vi "GUI.vi"() -> ()   [LabVIEW 2021]
panel:
  in  "Connection Type":u16(ring) items=["USB", "Ethernet"]
  in  "U6 Address":string="192.168.1.199"
  out "POWER\nDISCONNECTED":bool
  in  "?":bool
  in  "SV6":bool
  in  "SV5":bool
  in  "SV4":bool
  in  "START/STOP DATA LOGGING":bool
  in  "SHUTOFF POWER":bool
  in  "SHUTDOWN\nAPPROVE":bool
  in  "SV3":bool
  in  "SV2":bool
  in  "SV1":bool
  in  "SV0":bool
  out "ABORT\nACTIVATED":bool
  out "OVER TEMPERATURE":bool
  out "OVER\nPRESSURE":bool
  in  "GUITabs":T1(tab) caption="Tab Control"
  out "N2O Runtank [g/s]":i16(slide) scale=0.0..100.0
  out "Ethanol Runtank [g/s]":i16(slide) scale=0.0..100.0
  out "?":bool
  out "?":bool
  out "?":bool
  out "LabJack Supply Voltage":dbl(slide) scale=0.0..5.0
  out "Solenoid Supply Voltage":dbl(slide) scale=0.0..14.0
  out "Relay Supply Voltage":dbl(slide) scale=0.0..5.0
  out "PT3: Chamber Pressure [psig]":u16(knob) scale=0.0..500.0
  in  "Arm Button":bool
  in  "Fire Button":bool
  out "DEADMAN\nSWITCH":bool
  out "TC1: N2O Temp [°C]":i16(slide) scale=-270.0..370.0
  out "TC2: Chamber Temp [°C]":i16(slide) scale=-270.0..1260.0
  out "PT1: N2O Pressure [psig]":u16(knob) scale=0.0..1000.0
  out "PT2: Ethenol Pressure [psig]":u16(knob) scale=0.0..1000.0
  out "?":bool
  out "?":bool
  out "Thrust Reading [N]":dbl(slide) scale=0.0..200.0
  in  "Dry Test Run":bool
  in  "Valve\nDiagnostic":bool
  in  "Device\nDiagnostic":bool
  out "?":bool
  out "?":bool
  out "?":bool
  out "?":bool
  out "?":bool
  out "?":bool
  out "?":bool
  out "?":bool
  out "?":bool
  out "?":bool
  out "?":bool
  out "?":bool
  out "?":bool
  in  "S: NC/NO 7":bool
  in  "SV0 Pin":u16(ring)=8 items=["FIO0", "FIO1", "FIO2", "FIO3", "FIO4", "FIO5", "FIO6", "FIO7", "EIO0", "EIO1", "EIO2", "EIO3", "EIO4", "EIO5", "EIO6", "EIO7", "CIO0", "CIO1", "CIO2", "CIO3", "MIO0", "MIO1", "MIO2"]
  in  "SV1":u16(ring)=9 items=["FIO0", "FIO1", "FIO2", "FIO3", "FIO4", "FIO5", "FIO6", "FIO7", "EIO0", "EIO1", "EIO2", "EIO3", "EIO4", "EIO5", "EIO6", "EIO7", "CIO0", "CIO1", "CIO2", "CIO3", "MIO0", "MIO1", "MIO2"]
  in  "SV3 Pin":u16(ring)=11 items=["FIO0", "FIO1", "FIO2", "FIO3", "FIO4", "FIO5", "FIO6", "FIO7", "EIO0", "EIO1", "EIO2", "EIO3", "EIO4", "EIO5", "EIO6", "EIO7", "CIO0", "CIO1", "CIO2", "CIO3", "MIO0", "MIO1", "MIO2"]
  in  "SV2 Pin":u16(ring)=10 items=["FIO0", "FIO1", "FIO2", "FIO3", "FIO4", "FIO5", "FIO6", "FIO7", "EIO0", "EIO1", "EIO2", "EIO3", "EIO4", "EIO5", "EIO6", "EIO7", "CIO0", "CIO1", "CIO2", "CIO3", "MIO0", "MIO1", "MIO2"]
  in  "SV6 Pin":u16(ring)=14 items=["FIO0", "FIO1", "FIO2", "FIO3", "FIO4", "FIO5", "FIO6", "FIO7", "EIO0", "EIO1", "EIO2", "EIO3", "EIO4", "EIO5", "EIO6", "EIO7", "CIO0", "CIO1", "CIO2", "CIO3", "MIO0", "MIO1", "MIO2"]
  in  "SV5 Pin":u16(ring)=13 items=["FIO0", "FIO1", "FIO2", "FIO3", "FIO4", "FIO5", "FIO6", "FIO7", "EIO0", "EIO1", "EIO2", "EIO3", "EIO4", "EIO5", "EIO6", "EIO7", "CIO0", "CIO1", "CIO2", "CIO3", "MIO0", "MIO1", "MIO2"]
  in  "SV4 Pin":u16(ring)=12 items=["FIO0", "FIO1", "FIO2", "FIO3", "FIO4", "FIO5", "FIO6", "FIO7", "EIO0", "EIO1", "EIO2", "EIO3", "EIO4", "EIO5", "EIO6", "EIO7", "CIO0", "CIO1", "CIO2", "CIO3", "MIO0", "MIO1", "MIO2"]
  in  "S: NC/NO 6":bool
  in  "S: NC/NO 5":bool
  in  "S: NC/NO 4":bool
  in  "S: NC/NO 3":bool
  in  "S: NC/NO 2":bool=TRUE
  in  "S: NC/NO":bool=TRUE
  in  "R: NC/NO 7":bool=TRUE
  in  "R: NC/NO 6":bool=TRUE
  in  "R: NC/NO 5":bool=TRUE
  in  "R: NC/NO 4":bool=TRUE
  in  "R: NC/NO 3":bool=TRUE
  in  "R: NC/NO 2":bool=TRUE
  in  "R: NC/NO":bool=TRUE
  in  "?":bool
  in  "TC1 Type":u16(ring)=7 items=["B", "E", "J", "K", "N", "R", "S", "T"]
  in  "TC2 Type":u16(ring)=3 items=["B", "E", "J", "K", "N", "R", "S", "T"]
  in  "TC1 +Channel":u16
  in  "TC2 -Channel":u16=3
  in  "TC2 +Channel":u16=2
  in  "TC1 -Channel":u16=1
  in  "PT2 Pin":u16=6
  in  "PT1 Pin":u16=8
  in  "PT3 Pin":u16=4
  in  "LP1 Pin":u16=10
  in  "k":dbl=2000.0
  # "ABORT STATUS"
  # "MANUAL DATA CONTROL"
  # "OVERRIDE SYSTEM POWER"
  # "LABJACK CONNECTION"
  # "LINE & CHAMBER STATUS"
  # "HIL TEST PARAMETERS"
  # "SYSTEM FIRE OPERATION"
  # "SYSTEM TEST SEQUENCE"
  # "THRUST STATUS"
  # "RUNTANK STATUS"
  # "SYSTEM ERROR CALLSTACK"
  # "DATA LOGGING"
  # "PRESSURE TRANSMITTER SETTINGS"
  # "THERMOCOUPLE SETTINGS"
  # "SOLENOID VALVE & RELAY SETTINGS"
  # "CALIBRATION SETTINGS"
  # "LINEAR POTENTIOMETER SETTINGS"
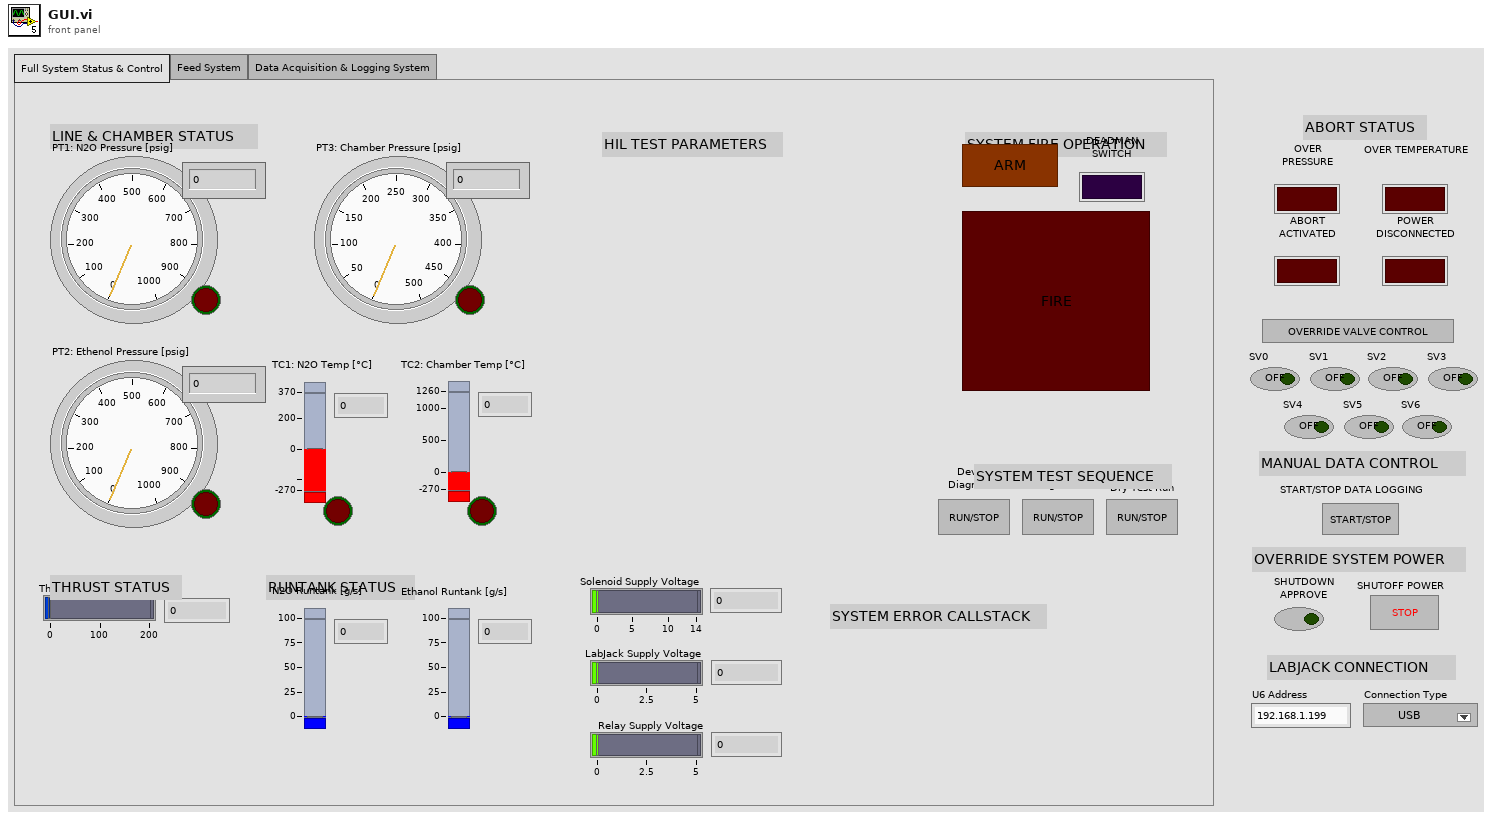
[diagram p1: front panel]
types:
  T1 = enum32{"Full System Status & Control", "Feed System", "Data Acquisition & Logging System"}
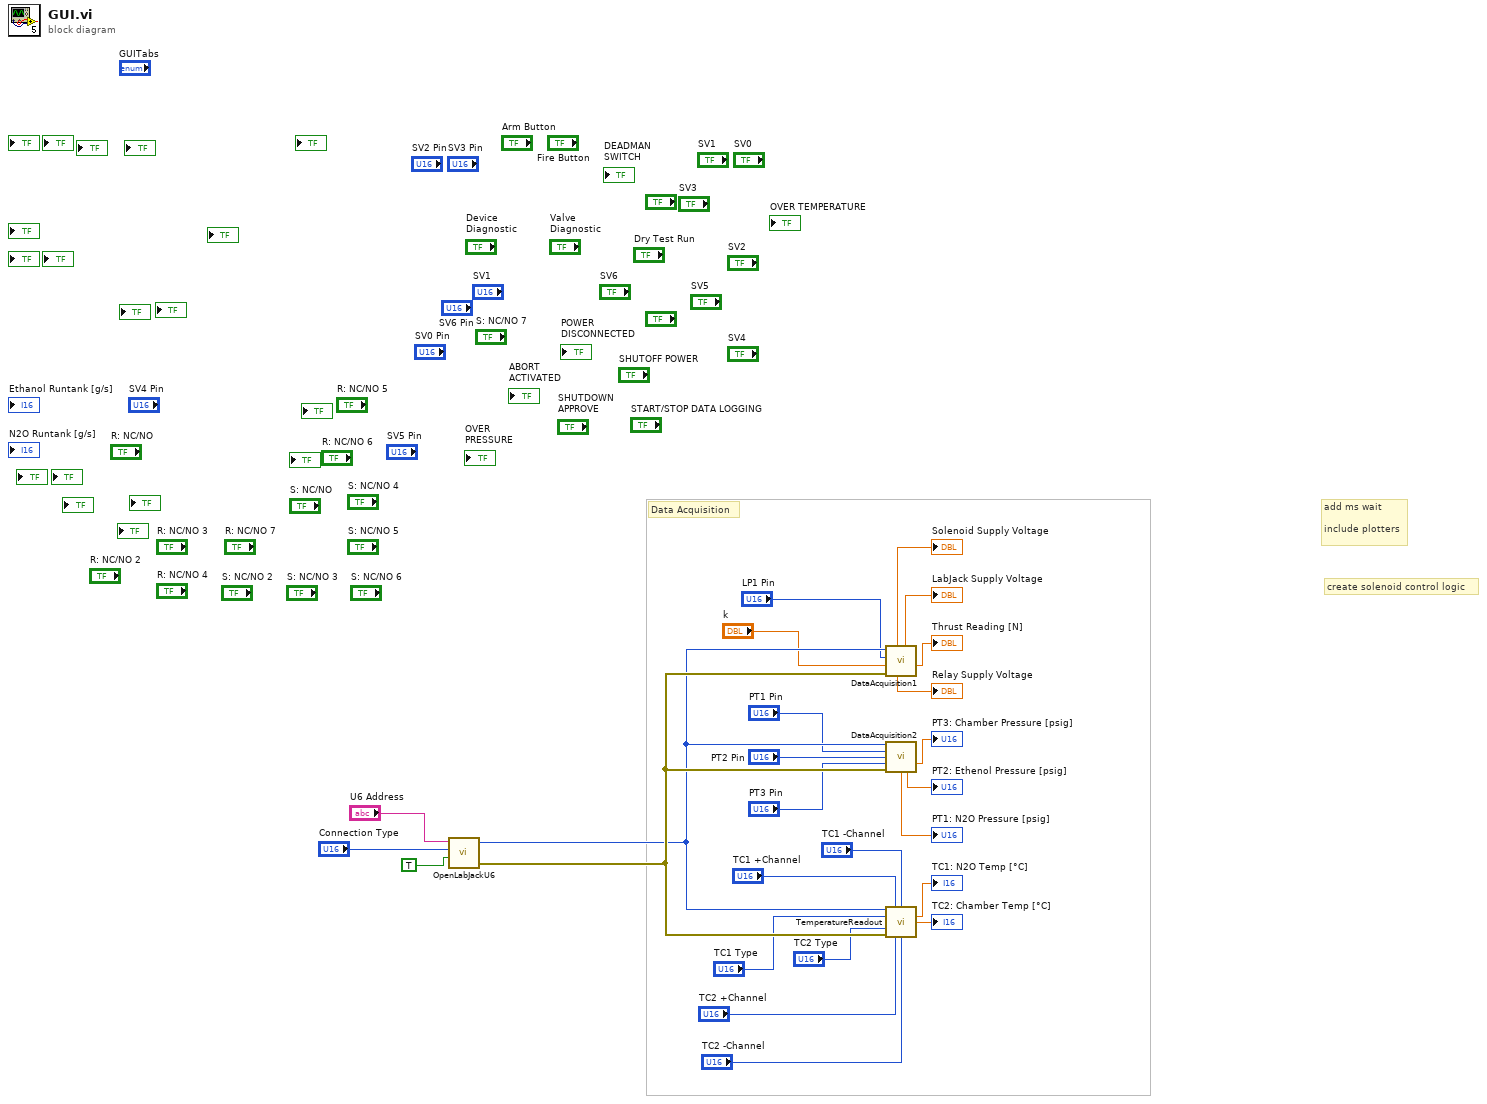
[diagram p0: block diagram]
diagram:
  # "create solenoid control logic"
  # "add ms wait\n\ninclude plotters"
  # "Data Acquisition"
  n1 = call "OpenLabJackU6.vi"("Select First Found"=TRUE, "Connection Type"="Connection Type", "U6 Address"="U6 Address") -> ("error out"=w23:errorcluster, "Handle"=w22:i32)  [unwired: 1 in, 1 out]
  n2 = call "DataAcquisition1.vi"("error in"=w23, "k"="k", "LP1 Pin"="LP1 Pin", "Handle In"=w22) -> ("Thrust Reading [Newton]"=→"Thrust Reading [N]":dbl, "LabJack Supply Voltage"=→"LabJack Supply Voltage":dbl, "Relay Supply Voltage"=→"Relay Supply Voltage":dbl, "Solenoid Supply Voltage"=→"Solenoid Supply Voltage":dbl)  [unwired: 3 out]
  n3 = call "DataAcquisition2.vi"("Handle In"=w22, "PT1 Pin"="PT1 Pin", "PT2 Pin"="PT2 Pin", "PT3 Pin"="PT3 Pin", "error in"=w23) -> ("PT3 Pressure Reading"=→"PT3: Chamber Pressure [psig]":dbl, "PT1 Pressure Reading"=→"PT1: N2O Pressure [psig]":dbl, "PT2 Pressure Reading"=→"PT2: Ethenol Pressure [psig]":dbl)  [unwired: 2 in, 6 out]
  n4 = call "TemperatureReadout.vi"("Handle In"=w22, "TC1 +Channel"="TC1 +Channel", "TC1 -Channel"="TC1 -Channel", "TC1 Type"="TC1 Type", "TC2 Type"="TC2 Type", "error in"=w23, "TC2 +Channel"="TC2 +Channel", "TC2 -Channel"="TC2 -Channel") -> ("TC1 Temperature (Deg C)"=→"TC1: N2O Temp [°C]":dbl, "TC2 Temperature (Deg C)"=→"TC2: Chamber Temp [°C]":dbl)  [unwired: 1 in, 5 out]
